vi "GEOM_RestoreAmplifiersOrder.vi"(9 "sorted amps":cluster{"number":i32, i32, i32}[](array[cluster]), 10 "orig amplifiers":T1[](array[typedef]) {"fliped" items=["none", "horizontal", "vertical"]; "type" items=["LL", "LR", "UL", "UR"]}) -> (2 "restored order":cluster{"number":i32, i32, i32}[](array[cluster]))   [LabVIEW 2016]
uses:
  GEOM_Amplifier.ctl
  GEOM_AmpType.ctl
  GEOM_ROI.ctl
  GEOM_Coords.ctl
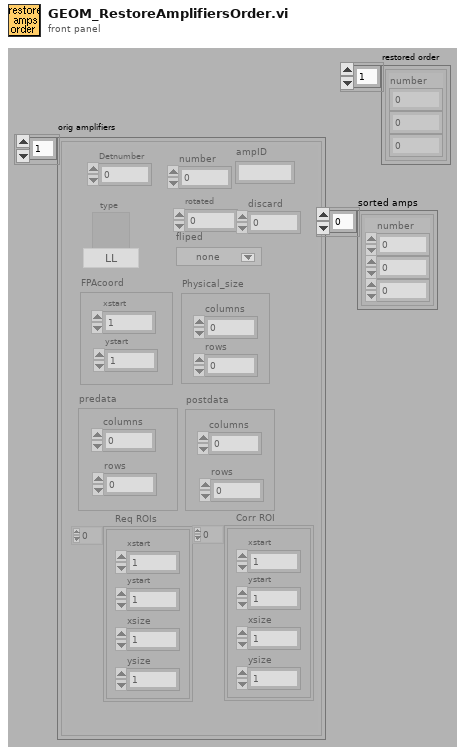
[diagram p1: front panel]
types:
  T1 = typedef "GEOM_Amplifier.ctl" = cluster{"number":i32, "type":T2, "rotated":i16, "fliped":u16, "FPAcoord":cluster{"xstart":i32, "ystart":i32}, "Physical_size":cluster{"columns":i32, "rows":i32}, "predata":cluster{"columns":i32, "rows":i32}, "postdata":cluster{"columns":i32, "rows":i32}, "Req ROIs":T3, "Corr ROI":T3, "Detnumber":i32, "ampID":string, "discard":i32}
  T2 = typedef "GEOM_AmpType.ctl" = u16
  T3 = typedef "GEOM_ROI.ctl" = T4[]
  T4 = typedef "GEOM_Coords.ctl" = cluster{"xstart":u32, "ystart":u32, "xsize":u32, "ysize":u32}
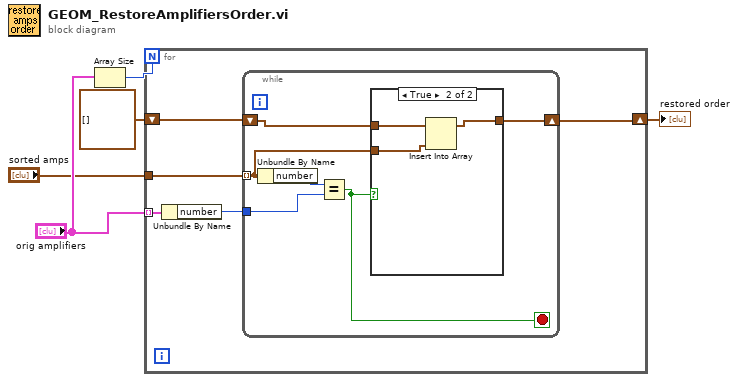
[diagram p0: block diagram]
diagram:
  n1 = Array Size(array="orig amplifiers") -> (size(s)=w5:i32)
  n2 = for {
    N: w5 -> [_]
    tunnel: "orig amplifiers" -> [w10] mode=indexing
    tunnel: "sorted amps" -> [w9]
    shift-right: [w7] -> w1
    shift-left: cluster{"number":i32, i32, i32}[] [] -> [w6]
    n3 = Unbundle By Name(w10) -> ("number"=w8:i32)
    n4 = while {
      tunnel: w9 -> [w13] mode=indexing
      tunnel: w8 -> [w15]
      shift-right: [w12] -> w7
      shift-left: w6 -> [w11]
      stop <- w14 stop-if-true
      n5 = Unbundle By Name(w13) -> ("number"=w16:i32)
      n6 = Equal?(x=w16, y=w15) -> (x = y?=w14:bool)
      n7 = case shown="True" w14 {
        tunnel: w13 -> [_ w20]
        tunnel: [w17 w19] -> w12
        tunnel: w11 -> [w17 w18]
        frame False {
        }
        frame True {
          n8 = Insert Into Array(array=w18, new element=w20) -> (w19:cluster{"number":i32, i32, i32}[])  [unwired: 1 in]
        }
      }
    }
  }
  "restored order" <- w1
